vi "Is Module Running.vi"(8 "error in (no error)":errorcluster, 11 "VI reference in":refnum<vi>) -> (0 "error out":errorcluster, 1 "Execution:State":T1(ring), 2 "Is Running?":bool, 3 "VI reference out":refnum<vi>)   [LabVIEW 2020, in "Controller.lvlib" / "Controller.lvclass"]
uses:
  Controller.lvclass
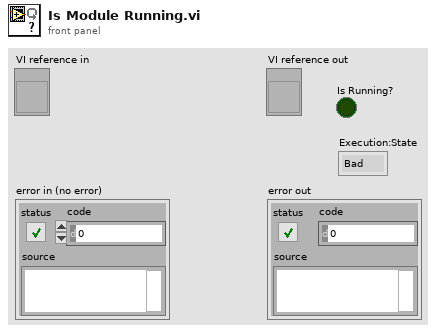
[diagram p1: front panel]
types:
  T1 = enum32{"Bad", "Idle", "Run top level", "Running"}
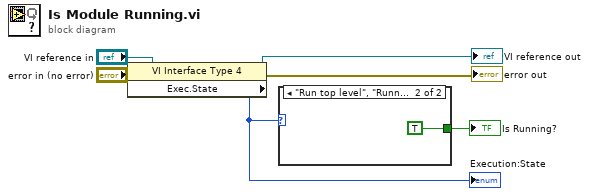
[diagram p0: block diagram]
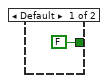
[diagram p2: hidden frame]
diagram:
  n1 = property class="VI Interface Type 4"(reference="VI reference in", error in="error in (no error)") -> (reference out=→"VI reference out":refnum<vi>, error out=→"error out":errorcluster, "Exec.State"=w6:T1)
  "Execution:State" <- w6
  n2 = case shown="\"Run top level\", \"Running\"" w6 {
    tunnel: [FALSE TRUE] -> w2
    frame Default {
    }
    frame "Run top level", "Running" {
    }
  }
  "Is Running?" <- w2
